vi "Actor Core.vi"(8 "error in":errorcluster, 11 "TRExperimentsRaw in":refnum<class "Samples.lvclass">) -> (0 "error out":errorcluster, 3 "Actor out":refnum<class "Actor.lvclass">)   [LabVIEW 2020, in "Forms.lvlib" / "Samples.lvclass"]
doc: "The user interface for this panel.\n\n----\nPlease see the following web address for additional documentation and tutorial information:\nhttp://www.mooregoodideas.com/mgi-panel-manager/\n\nAuthor: Derek Trepanier\n\nCopyright (c) 2018, Moore Good Ideas, Inc.\n\nAll rights reserved.\n\nRedistribution and use in source and binary forms, with or without modification, are permitted provided that the following conditions are met:\n\n * Redistributions of source code must retain the above copyright notice, this list of conditions and the following disclaimer.\n * Redistributions in binary form must reproduce the above copyright notice, this list of conditions and the following disclaimer in the documentation and/or other materials provided with the distribution.\n * Neither the name of Moore Good Ideas, Inc. nor the names of its contributors may be used to endorse or promote products derived from this software without specific prior written permission.\n\nTHIS SOFTWARE IS PROVIDED BY THE COPYRIGHT HOLDERS AND CONTRIBUTORS \"AS IS\" AND ANY EXPRESS OR IMPLIED WARRANTIES, INCLUDING, BUT NOT LIMITED TO, THE IMPLIED WARRANTIES OF MERCHANTABILITY AND FITNESS FOR A PARTICULAR PURPOSE ARE DISCLAIMED. IN NO EVENT SHALL THE COPYRIGHT OWNER OR CONTRIBUTORS BE LIABLE FOR ANY DIRECT, INDIRECT, INCIDENTAL, SPECIAL, EXEMPLARY, OR CONSEQUENTIAL DAMAGES (INCLUDING, BUT NOT LIMITED TO, PROCUREMENT OF SUBSTITUTE GOODS OR SERVICES; LOSS OF USE, DATA, OR PROFITS; OR BUSINESS INTERRUPTION) HOWEVER CAUSED AND ON ANY THEORY OF LIABILITY, WHETHER IN CONTRACT, STRICT LIABILITY, OR TORT (INCLUDING NEGLIGENCE OR OTHERWISE) ARISING IN ANY WAY OUT OF THE USE OF THIS SOFTWARE, EVEN IF ADVISED OF THE POSSIBILITY OF SUCH DAMAGE."
uses:
  Samples.lvclass
  C:/Users/User/Desktop/Raman Program/Database OOP/forms AF/Form Controller/Panel Form Controller.lvclass
  <vilib>/ActorFramework/Actor/Actor.lvclass
  Text Field Info.ctl
  Numeric Field Info.ctl
  FK Ring Field Info.ctl
  FK Ring Info.ctl
  Open Form.lvclass
  C:/Users/User/Desktop/Raman Program/Database OOP/source/Button/Button.lvclass
  Users.lvclass
  Sample Chemical Formula.lvclass
  Panel Form Controller.lvclass/Panel Form Controller.ctl
  Constructor by Info Cluster Text.vi
  Constructor by Info Cluster Numeric.vi
  Constructor by Info Cluster FK Ring.vi
  Panel Form Controller.lvclass
  Field.lvclass
panel:
  in  "Add Formula":bool
  in  "Add User":bool
  in  "Chemical Formula":u16(ring)
  in  "User":u16(ring)
  in  "Doping Density (%)":dbl
  in  "Display Name":string
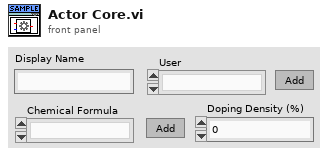
[diagram p1: front panel]
types:
  T1 = typedef "Numeric Field Info.ctl" = cluster{"Ctl Refnum":refnum<vi>, "Table":string, "Column":string}
  T2 = typedef "FK Ring Field Info.ctl" = cluster{"Ctl Refnum":refnum<vi>, "FK Table":string, "FK Column":string, "FK Ring Info":T3}
  T3 = typedef "FK Ring Info.ctl" = cluster{"PK Table":string, "PK Column":string, "PK Display Column":string}
  T4 = typedef "Panel Form Controller.lvlib/Builder Cluster.ctl" = cluster{"Field Map":map{string, refnum<class "Field.lvclass">}, "Button Map":map{string, refnum<class "Button.lvclass">}, "Initialized Field":refnum<class "Field.lvclass">, "VI Ctrl Array":refnum<vi>[]}
  T5 = typedef "Text Field Info.ctl" = cluster{"Ctl Refnum":refnum<vi>, "Table":string, "Column":string}
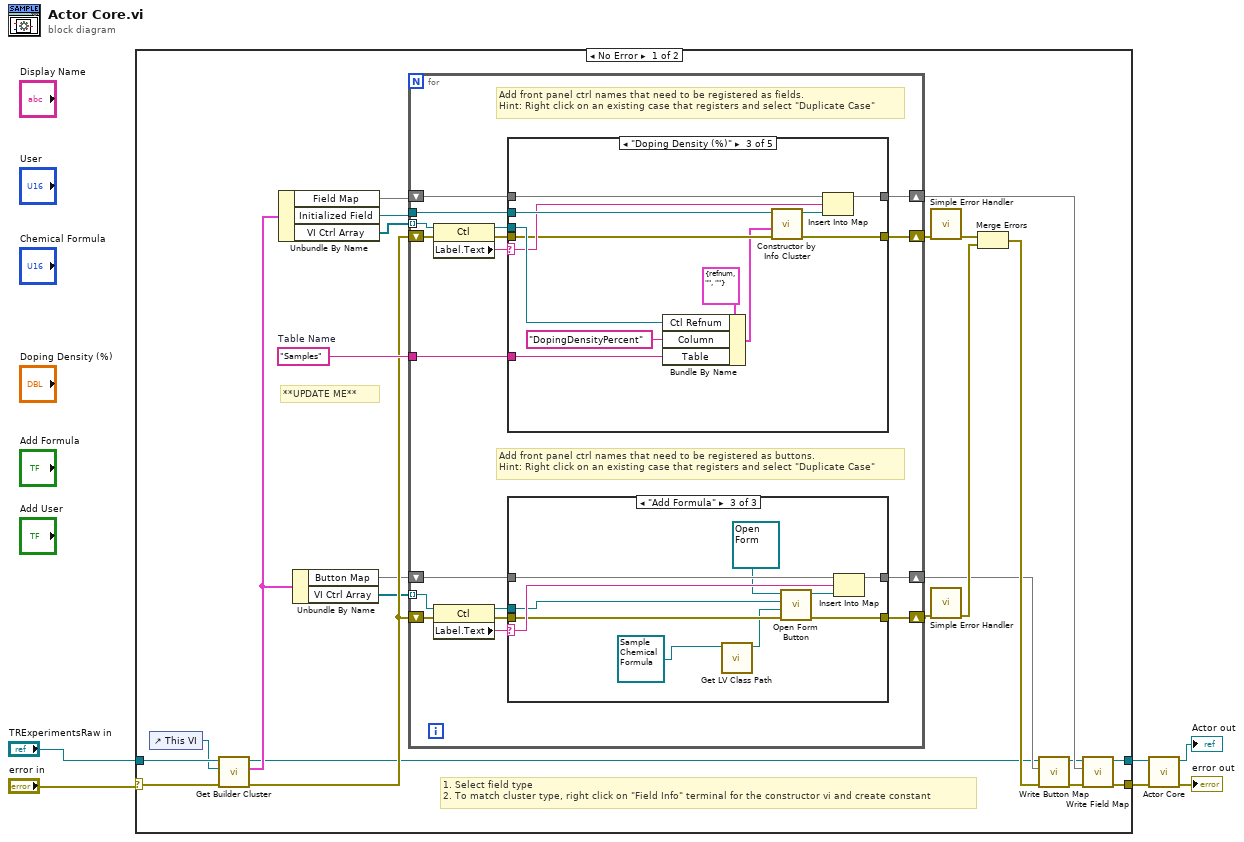
[diagram p0: block diagram]
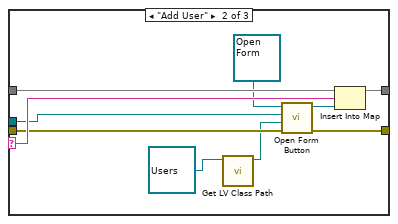
[diagram p3: hidden frame]
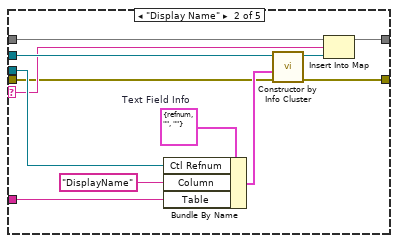
[diagram p5: hidden frame]
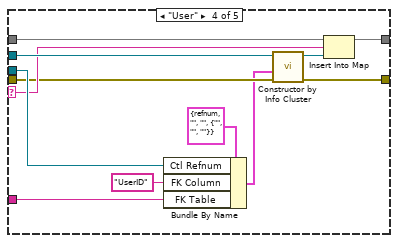
[diagram p6: hidden frame]
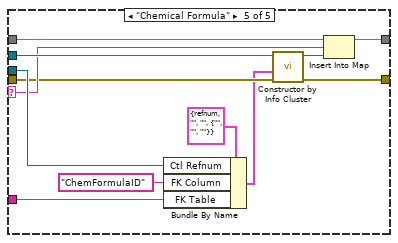
[diagram p7: hidden frame]
diagram:
  n1 = case shown="No Error" "error in" {
    selector: "error in" -> [w10 w121]
    tunnel: "TRExperimentsRaw in" -> [w27 w120]
    tunnel: [w9 w121] -> w3
    tunnel: [w8 w120] -> w4
    frame No Error {
      w29 = "Samples"  # Table Name
      # "1. Select field type\n2. To match cluster type, right click on \"Field Info\" terminal for the constructor vi and create constant"
      # "**UPDATE ME**"
      n2 = control-ref of="This VI"() -> (w7:refnum<vi>)
      n3 = call "Get Builder Cluster.vi"("error in (no error)"=w10, "VI Refnum"=w7, "Panel Form Controller in"=w27) -> ("error out"=w22:errorcluster, "Builder Cluster"=w20:T4, "Panel Form Controller out"=w11:refnum<class "Samples.lvclass">)  [unwired: 6 in]
      n4 = Unbundle By Name(w20) -> ("Field Map"=w26:map{string, refnum<class "Field.lvclass">}, "Initialized Field"=w25:refnum<class "Field.lvclass">, "VI Ctrl Array"=w24:refnum<vi>[])
      n5 = Unbundle By Name(w20) -> ("Button Map"=w19:map{string, refnum<class "Button.lvclass">}, "VI Ctrl Array"=w18:refnum<vi>[])
      n6 = for {
        tunnel: w24 -> [w47] mode=indexing
        tunnel: w25 -> [w45]
        tunnel: w29 -> [w44]
        shift-right: [w38] -> w23
        shift-left: w26 -> [w39]
        shift-right: [w43] -> w28
        shift-left: w22 -> [w42]
        shift-right: [w37] -> w21
        shift-left: w22 -> [w36]
        tunnel: w18 -> [w34] mode=indexing
        shift-right: [w31] -> w12
        shift-left: w19 -> [w32]
        # "Add front panel ctrl names that need to be registered as buttons.\nHint: Right click on an existing case that registers and select \"Duplicate Case\""
        # "Add front panel ctrl names that need to be registered as fields.\nHint: Right click on an existing case that registers and select \"Duplicate Case\""
        n7 = property class="Ctl"(reference=w47, error in=w42) -> (reference out=w46:refnum<vi>, error out=w41:errorcluster, "Label.Text"=w40:string)
        n8 = property class="Ctl"(reference=w34, error in=w36) -> (reference out=w33:refnum<vi>, error out=w35:errorcluster, "Label.Text"=w30:string)
        n9 = case shown="\"Doping Density (%)\"" w40 {
          selector: w40 -> [_ w75 w89 w101 w113]
          tunnel: w46 -> [_ w80 w94 w106 w118]
          tunnel: w45 -> [_ w83 w95 w107 w119]
          tunnel: w44 -> [_ w79 w93 w105 w117]
          tunnel: w39 -> [w71 w78 w92 w104 w116]
          tunnel: [w71 w77 w91 w103 w115] -> w38
          tunnel: [w70 w74 w88 w100 w112] -> w43
          tunnel: w41 -> [w70 w73 w87 w99 w111]
          frame Default {
          }
          frame "Display Name" {
            w82 = T5 {"Ctl Refnum"=refnum, "Table"="", "Column"=""}  # Text Field Info
            n10 = Bundle By Name(cluster=w82, "Ctl Refnum"=w80, "Column"="DisplayName", "Table"=w79) -> (w81:T5)
            n11 = call-poly "Constructor by Info Cluster.vi"("error in (no error)"=w73, "Text Field Info"=w81, "Field in"=w83) -> ("error out"=w74:errorcluster, "Field out"=w76:refnum<class "Field.lvclass">)  [unwired: 7 in]
            n12 = Insert Into Map(map in=w78, key=w75, value=w76) -> (map out=w77:map{string, refnum<class "Field.lvclass">})  [unwired: 2 out]
          }
          frame "Doping Density (%)" {
            n13 = Bundle By Name(cluster=T1 {"Ctl Refnum"=refnum, "Table"="", "Column"=""} ("Numeric Field Info"), "Ctl Refnum"=w94, "Column"="DopingDensityPercent", "Table"=w93) -> (w84:T1)
            n14 = call-poly "Constructor by Info Cluster.vi"("error in (no error)"=w87, "Numeric Field Info"=w84, "Field in"=w95) -> ("error out"=w88:errorcluster, "Field out"=w90:refnum<class "Field.lvclass">)  [unwired: 7 in]
            n15 = Insert Into Map(map in=w92, key=w89, value=w90) -> (map out=w91:map{string, refnum<class "Field.lvclass">})  [unwired: 2 out]
          }
          frame "User" {
            n16 = Bundle By Name(cluster=T2 {"Ctl Refnum"=refnum, "FK Table"="", "FK Column"="", "FK Ring Info"={"PK Table"="", "PK Column"="", "PK Display Column"=""}} ("FK Ring Field Info"), "Ctl Refnum"=w106, "FK Column"="UserID" ("Column"), "FK Table"=w105) -> (w96:T2)
            n17 = call-poly "Constructor by Info Cluster.vi"("error in (no error)"=w99, "FK Ring Field Info"=w96, "Field in"=w107) -> ("error out"=w100:errorcluster, "Field out"=w102:refnum<class "Field.lvclass">)  [unwired: 7 in]
            n18 = Insert Into Map(map in=w104, key=w101, value=w102) -> (map out=w103:map{string, refnum<class "Field.lvclass">})  [unwired: 2 out]
          }
          frame "Chemical Formula" {
            n19 = Bundle By Name(cluster=T2 {"Ctl Refnum"=refnum, "FK Table"="", "FK Column"="", "FK Ring Info"={"PK Table"="", "PK Column"="", "PK Display Column"=""}} ("FK Ring Field Info"), "Ctl Refnum"=w118, "FK Column"="ChemFormulaID" ("Column"), "FK Table"=w117) -> (w108:T2)
            n20 = call-poly "Constructor by Info Cluster.vi"("error in (no error)"=w111, "FK Ring Field Info"=w108, "Field in"=w119) -> ("error out"=w112:errorcluster, "Field out"=w114:refnum<class "Field.lvclass">)  [unwired: 7 in]
            n21 = Insert Into Map(map in=w116, key=w113, value=w114) -> (map out=w115:map{string, refnum<class "Field.lvclass">})  [unwired: 2 out]
          }
        }
        n22 = case shown="\"Add Formula\"" w30 {
          selector: w30 -> [_ w57 w67]
          tunnel: w33 -> [_ w55 w65]
          tunnel: [w49 w53 w63] -> w37
          tunnel: w35 -> [w49 w54 w64]
          tunnel: w32 -> [w48 w59 w69]
          tunnel: [w48 w58 w68] -> w31
          frame Default {
          }
          frame "Add User" {
            n23 = call <vilib>:"Get LV Class Path.vi"("object"=refnum<class "Users.lvclass"> refnum ("Forms.lvlib:Users.lvclass")) -> ("class path"=w51:path)  [unwired: 9 in, 1 out]
            n24 = call "Open Form Button.vi"("error in (no error)"=w54, "Class Path"=w51, "Ctl Refnum"=w55, "Open Form in"=refnum<class "Open Form.lvclass"> refnum) -> ("error out"=w53:errorcluster, "Open Form out"=w56:refnum<class "Open Form.lvclass">)  [unwired: 6 in]
            n25 = Insert Into Map(map in=w59, key=w57, value=w56) -> (map out=w58:map{string, refnum<class "Button.lvclass">})  [unwired: 2 out]
          }
          frame "Add Formula" {
            n26 = call <vilib>:"Get LV Class Path.vi"("object"=refnum<class "Sample Chemical Formula.lvclass"> refnum ("Forms.lvlib:Sample Chemical Formula.lvclass")) -> ("class path"=w61:path)  [unwired: 9 in, 1 out]
            n27 = call "Open Form Button.vi"("error in (no error)"=w64, "Class Path"=w61, "Ctl Refnum"=w65, "Open Form in"=refnum<class "Open Form.lvclass"> refnum) -> ("error out"=w63:errorcluster, "Open Form out"=w66:refnum<class "Open Form.lvclass">)  [unwired: 6 in]
            n28 = Insert Into Map(map in=w69, key=w67, value=w66) -> (map out=w68:map{string, refnum<class "Button.lvclass">})  [unwired: 2 out]
          }
        }
      }
      n29 = call <vilib>:"Simple Error Handler.vi"("error in (no error)"=w28) -> ("error out"=w16:errorcluster)  [unwired: 4 in, 4 out]
      n30 = call <vilib>:"Simple Error Handler.vi"("error in (no error)"=w21) -> ("error out"=w17:errorcluster)  [unwired: 4 in, 4 out]
      n31 = Merge Errors(w16, w17) -> (w15:errorcluster)
      n32 = call "Write Button Map.vi"("error in (no error)"=w15, "Button Map"=w12, "Panel Form Controller in"=w11) -> ("error out"=w14:errorcluster, "Panel Form Controller out"=w13:refnum<class "Samples.lvclass">)  [unwired: 7 in]
      n33 = call "Write Field Map.vi"("error in (no error)"=w14, "Field Map"=w23, "Panel Form Controller in"=w13) -> ("error out"=w9:errorcluster, "Panel Form Controller out"=w8:refnum<class "Samples.lvclass">)  [unwired: 7 in]
    }
    frame Error {
    }
  }
  n34 = call-parent "Actor Core.vi"("error in"=w3, "Panel Form Controller in"=w4) -> ("error out"=→"error out":errorcluster, "Actor out"=→"Actor out":refnum<class "Actor.lvclass">)  [unwired: 8 in]
